vi "start.vi"(8 "error in (no error)":errorcluster, 11 "AndorIKonAcquisitor in":refnum<class "AndorIKonAcquisitor.lvclass">) -> (0 "error out":errorcluster, 3 "AndorIKonAcquisitor out":refnum<class "AndorIKonAcquisitor.lvclass">)   [LabVIEW 2009, in "Hardware.lvlib" / "Channels.lvlib" / "AndorIKonAcquisitor.lvclass"]
uses:
  AndorIKonAcquisitor.lvclass
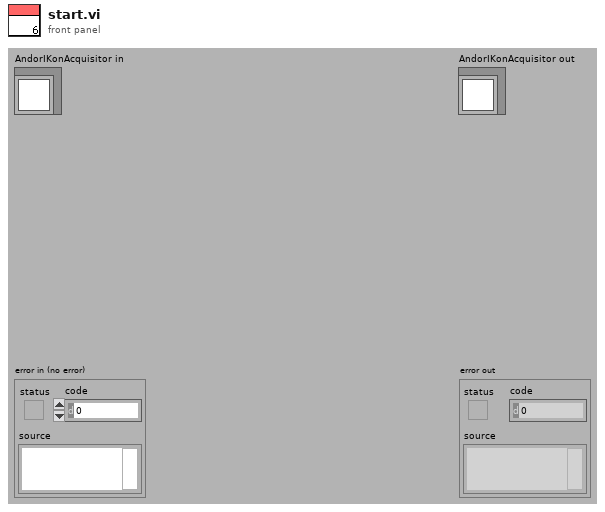
[diagram p1: front panel]
types:
  T1 = typedef "Error Code Enum typedef.ctl" = enum32{"N/A (0)", "DRV_ERROR_CODES", "DRV_SUCCESS", "DRV_VXDNOTINSTALLED", "DRV_ERROR_SCAN", "DRV_ERROR_CHECK_SUM", "DRV_ERROR_FILELOAD", "DRV_UNKNOWN_FUNC", "DRV_ERROR_VXD_INIT", "DRV_ERROR_ADDRESS", "DRV_ERROR_PAGELOCK", "DRV_ERROR_PAGEUNLOCK", "DRV_ERROR_BOARDTEST", "DRV_ERROR_ACK", "DRV_ERROR_UP_FIFO", "DRV_ERROR_PATTERN", "N/A (16)", "DRV_ACQUISITION_ERRORS", "DRV_ACQ_BUFFER", "DRV_ACQ_DOWNFIFO_FULL", "DRV_PROC_UNKONWN_INSTRUCTION", "DRV_ILLEGAL_OP_CODE", "DRV_KINETIC_TIME_NOT_MET", "DRV_ACCUM_TIME_NOT_MET", "DRV_NO_NEW_DATA", "N/A (25)", "DRV_SPOOLERROR", "N/A (27)", "N/A (28)", "N/A (29)", "N/A (30)", "N/A (31)", "N/A (32)", "DRV_TEMPERATURE_CODES", "DRV_TEMPERATURE_OFF", "DRV_TEMPERATURE_NOT_STABILIZED", "DRV_TEMPERATURE_STABILIZED", "DRV_TEMPERATURE_NOT_REACHED", "DRV_TEMPERATURE_OUT_RANGE", "DRV_TEMPERATURE_NOT_SUPPORTED", "DRV_TEMPERATURE_DRIFT", "N/A (41)", "N/A (42)", "N/A (43)", "N/A (44)", "N/A (45)", "N/A (46)", "N/A (47)", "N/A (48)", "DRV_GENERAL_ERRORS", "DRV_INVALID_AUX", "DRV_COF_NOTLOADED", "DRV_FPGAPROG", "DRV_FLEXERROR", "DRV_GPIBERROR", "N/A (55)", "N/A (56)", "N/A (57)", "N/A (58)", "N/A (59)", "N/A (60)", "N/A (61)", "N/A (62)", "N/A (63)", "DRV_DATATYPE", "DRV_DRIVER_ERRORS", "DRV_P1INVALID", "DRV_P2INVALID", "DRV_P3INVALID", "DRV_P4INVALID", "DRV_INIERROR", "DRV_COFERROR", "DRV_ACQUIRING", "DRV_IDLE", "DRV_TEMPCYCLE", "DRV_NOT_INITIALIZED", "DRV_P5INVALID", "DRV_P6INVALID", "DRV_INVALID_MODE", "DRV_INVALID_FILTER", "DRV_I2CERRORS", "DRV_I2CDEVNOTFOUND", "DRV_I2CTIMEOUT", "DRV_P7INVALID", "N/A (84)", "N/A (85)", "N/A (86)", "N/A (87)", "N/A (88)", "N/A (89)", "DRV_IOCERROR", "DRV_VRMVERSIONERROR"}
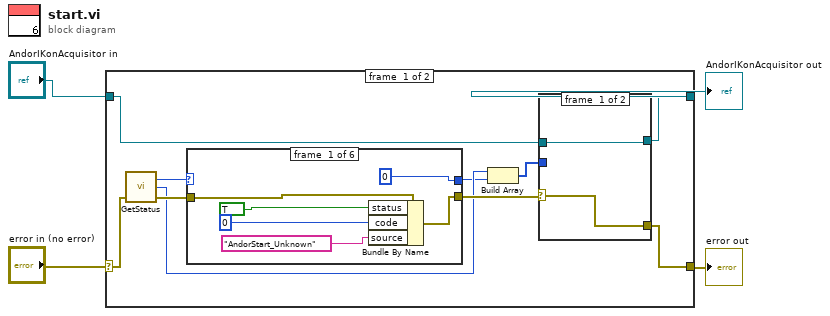
[diagram p0: block diagram]
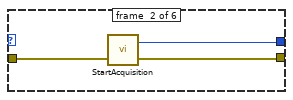
[diagram p2: hidden frame]
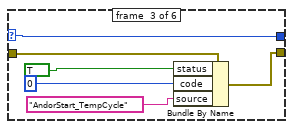
[diagram p3: hidden frame]
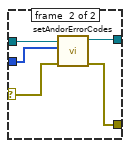
[diagram p7: hidden frame]
diagram:
  n1 = case shown="No Error" "error in (no error)" {
    selector: "error in (no error)" -> [w10 w44]
    tunnel: "AndorIKonAcquisitor in" -> [w13 w43]
    tunnel: [w12 w43] -> w2
    tunnel: [w11 w44] -> w1
    frame #0 {
      n2 = call <userlib>:"GetStatus.vi"("error in (no error)"=w10) -> ("error out"=w8:errorcluster, "DLL error code"=w7:u32, "status"=w5:T1)  [unwired: 2 in]
      n3 = case shown="\"DRV_IDLE\"" w5 {
        selector: w5 -> [_ _ w29 w31 w33 w35]
        tunnel: [0 w23 w29 w31 w33 w35] -> w6
        tunnel: [w15 w22 w24 w30 w32 w34] -> w14
        tunnel: w8 -> [w16 w21 w28 w30 w32 w34]
        frame #0 {
          n4 = Bundle By Name(cluster=w16, "status"=TRUE, "code"=0, "source"="AndorStart_Unknown") -> (w15:errorcluster)
        }
        frame #1 {
          n5 = call <userlib>:"StartAcquisition.vi"("error in (no error)"=w21) -> ("error out"=w22:errorcluster, "DLL error code"=w23:u32)  [unwired: 1 in]
        }
        frame #2 {
          n6 = Bundle By Name(cluster=w28, "status"=TRUE, "code"=0, "source"="AndorStart_TempCycle") -> (w24:errorcluster)
        }
        frame #3 {
        }
        frame #4 {
        }
        frame #5 {
        }
      }
      n7 = Build Array(w7, w6) -> (w9:u32[])
      n8 = case shown="Error" w14 {
        selector: w14 -> [w37 w41]
        tunnel: w13 -> [w36 w42]
        tunnel: [w36 w39] -> w12
        tunnel: [w37 w40] -> w11
        tunnel: w9 -> [_ w38]
        frame #0 {
        }
        frame #1 {
          n9 = call-dynamic "setAndorErrorCodes.vi"("error in (no error)"=w41, "Andor Error Codes"=w38, "AndorIKonAcquisitor.lvclass in"=w42) -> ("error out"=w40:errorcluster, "AndorIKonAcquisitor.lvclass out"=w39:refnum<class "AndorIKonAcquisitor.lvclass">)  [unwired: 7 in]
        }
      }
    }
    frame #1 {
    }
  }
  "error out" <- w1
  "AndorIKonAcquisitor out" <- w2
